vi "Global_Vision_CMDs.vi"() -> ()   [LabVIEW 2017, in "VisionHW.lvlib"]
uses:
  Systems/VisionHW Folder/VisionHW.lvlib
  TypeDefs/ENUM_Vision_Commands.ctl
panel:
  in  "Vision_Modes":T1=enum."ResetCamera"
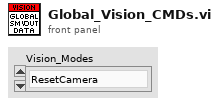
[diagram p1: front panel]
types:
  T1 = typedef "ENUM_Vision_Commands.ctl" = enum16{"Init", "NoOp", "ResetCamera", "VideoOn", "VideoOff", "CubeDetection", "RoadNavigation"}
diagram:
